vi "TURN_V2.vi"(0 "datain":string[](array[string])=["备注", "负载通道", "负载地址", "延时时间", "output max", "output min", "量测类型", "待测物板号"], 5 "HW CH Number":i32=4, 7 "Setup":string) -> (4 "REPORT INDECATE":string[][](array[string])=[["微安测试", "", "", "", ""], ["微安量测", "4", "0.000", "0.1", "NG"], ["微安量测", "4", "0.000", "0.1", "NG"], ["微安量测", "4", "0.000", "0.1", "NG"], ["微安量测", "4", "0.000", "0.1", "NG"]], 6 "ROW HEAD":string[](array[string]), 8 "PF":string[](array[string]), 10 "testData":string[](array[string]), 14 "数组":bool[](array[boolean]), 15 "Array":string[](array[string]))   [LabVIEW 2018]
uses:
  Subvi/Global.vi
panel:
  out "测试板数":i32=4
  # "[VoltageTest]\nExt.Name =2222222222;\nAddress =1;\nDelay Time =1;\nMAX.Spec =*;\nMin.Spec =2;\nTest Type =;\nRelayH_8Bit =0,0,0,0;\nRelayL_8Bit =0,0,0,0;\nStart board number =1;#"
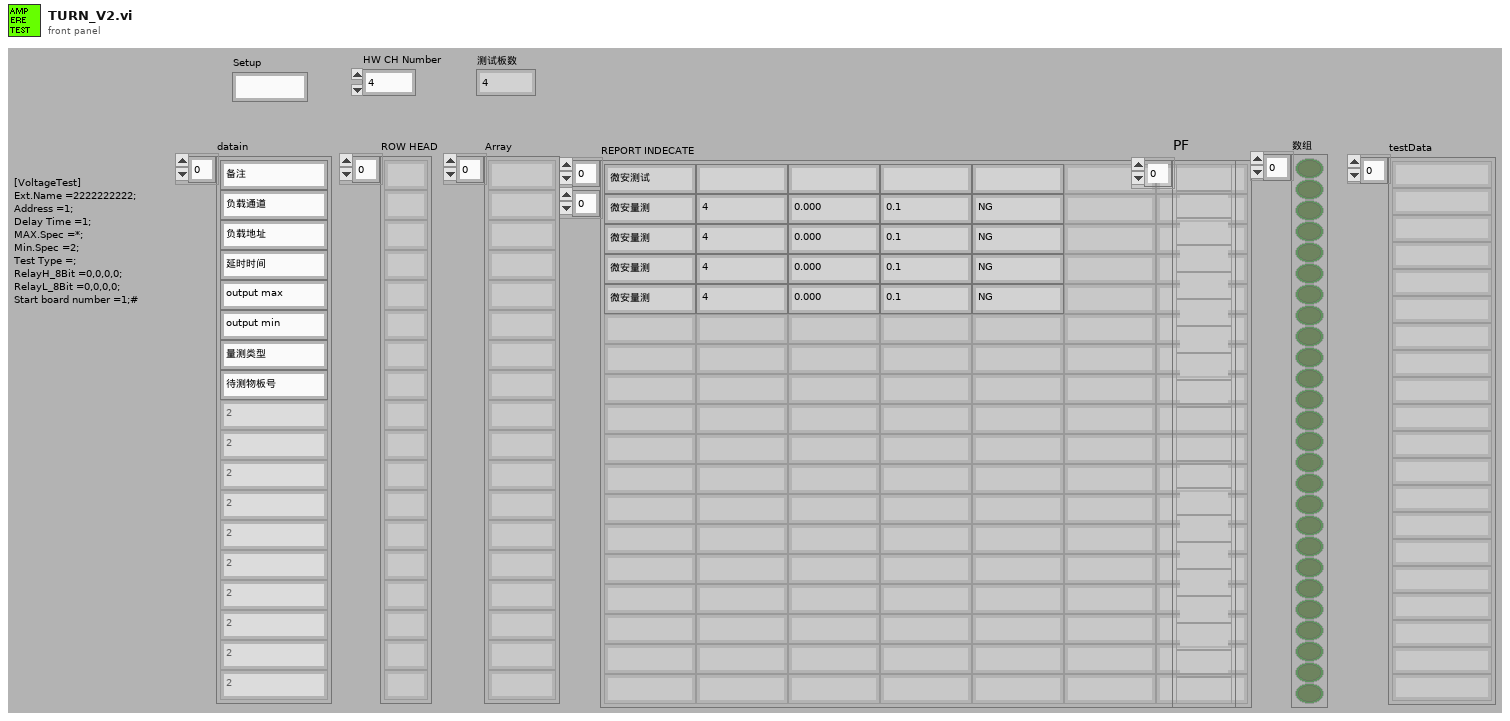
[diagram p1: front panel]
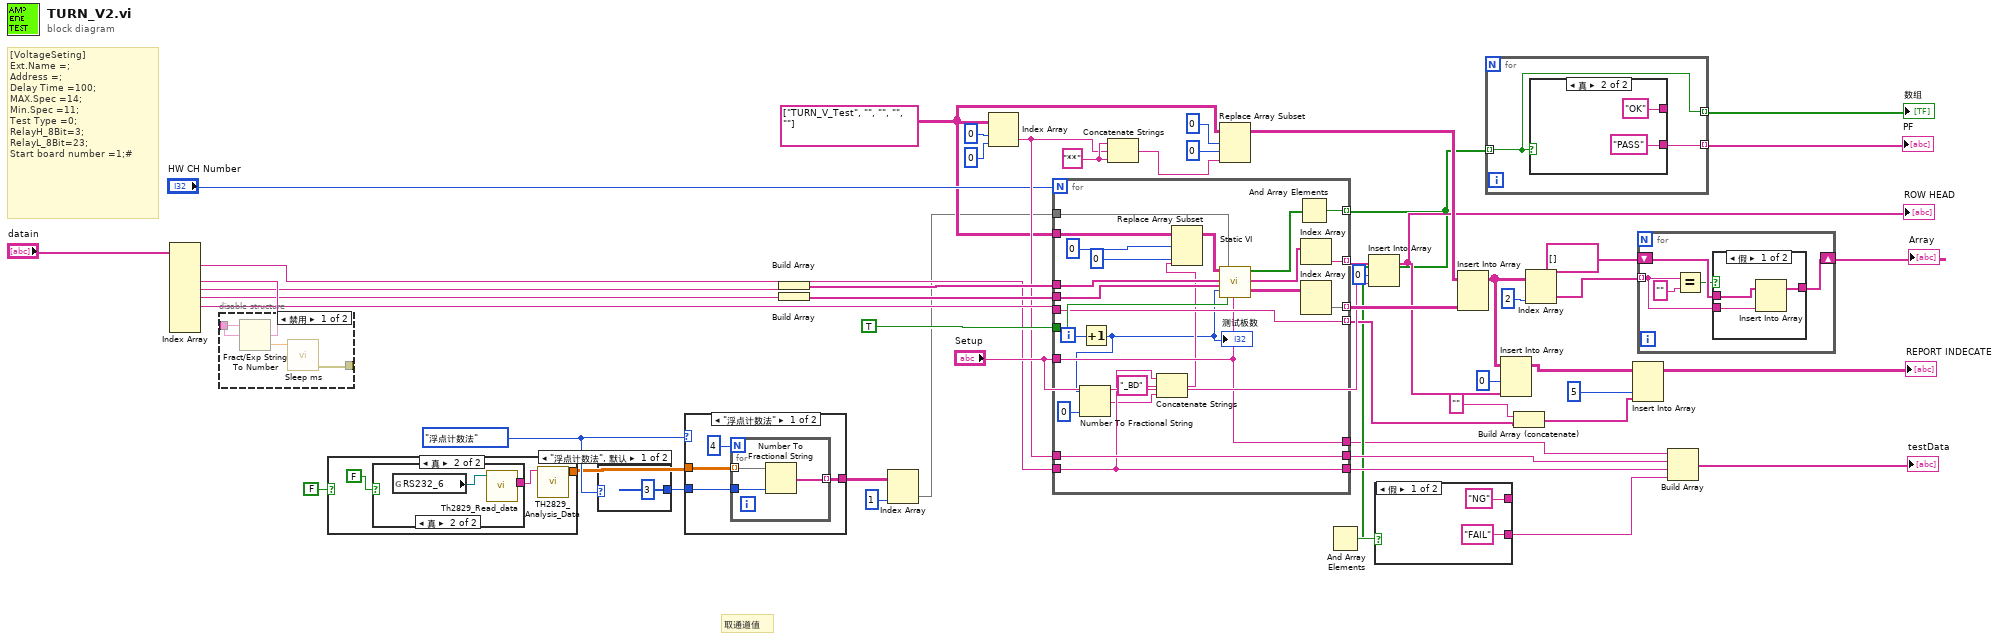
[diagram p0: block diagram]
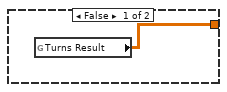
[diagram p2: hidden frame]
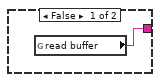
[diagram p3: hidden frame]
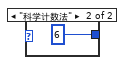
[diagram p4: hidden frame]
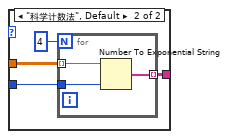
[diagram p5: hidden frame]
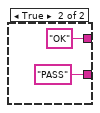
[diagram p7: hidden frame]
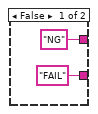
[diagram p8: hidden frame]
diagram:
  w6 = enum16{"浮点计数法", "科学计数法"}."浮点计数法" ("显示格式")
  w8 = string[][] [["TURN_V_Test", "", "", "", ""]]
  w43 = "**" ("字符串")
  # "取通道值"
  # "[VoltageSeting]\nExt.Name =;\nAddress =;\nDelay Time =100;\nMAX.Spec =14;\nMin.Spec =11;\nTest Type =0;\nRelayH_8Bit=3;\nRelayL_8Bit=23;\nStart board number =1;#"
  n1 = Index Array(array="datain") -> (element #1=w9:string, element #3=w46:string, element #4=w39:string, element #5=w38:string, element #6=w26:string)  [unwired: 9 in, 4 out]
  n2 = disable-structure shown="禁用" {
    disable-tunnel: w46 -> [w55 _]
    disable-tunnel: [w54 _] -> _
    frame Disabled {
      n3 = Fract/Exp String To Number(string=w55) -> (number=w53:dbl)  [unwired: 3 in, 1 out]
      n4 = call "Sleep ms.vi"("等待时间（毫秒）"=w53) -> ("error out"=w54:errorcluster)  [unwired: 10 in]
    }
    frame Enabled {
    }
  }
  n5 = case shown="真" FALSE {
    tunnel: [w56 w57] -> w5
    frame False {
      n6 = global read "Global.vi" "Turns Result"() -> (w56:sgl[][])
    }
    frame True {
      n7 = case shown="真" FALSE {
        tunnel: [w60 w62] -> w59
        frame False {
          n8 = global read "Global.vi" "read buffer"() -> (w60:string)
        }
        frame True {
          n9 = global read "Global.vi" "RS232_6"() -> (w61:refnum<visa-resource-name>)
          n10 = call "Th2829_Read_data.vi"("VISA资源名称"=w61) -> ("读取缓冲区"=w62:string)  [unwired: 9 in, 1 out]
        }
      }
      n11 = call "TH2829_Analysis_Data.vi"("字符串"=w59) -> ("Turns Result"=w57:sgl[][])  [unwired: 15 in, 3 out]
    }
  }
  n12 = case shown="\"浮点计数法\", 默认" w6 {
    tunnel: [i16 3 ("精度(6)") i16 6 ("精度(6)")] -> w7
    frame "浮点计数法", Default {
    }
    frame "科学计数法" {
    }
  }
  n13 = case shown="\"浮点计数法\"" w6 {
    tunnel: w5 -> [w67 w74]
    tunnel: [w66 w73] -> w4
    tunnel: w7 -> [w65 w72]
    frame "浮点计数法" {
      n14 = for {
        N: 4 -> [_]
        tunnel: w67 -> [w71] mode=indexing
        tunnel: [w70] -> w66 mode=indexing
        tunnel: w65 -> [w69]
        n15 = Number To Fractional String(number=w71, precision (6)=w69) -> (F-format string=w70:string[])  [unwired: 2 in]
      }
    }
    frame "科学计数法", Default {
      n16 = for {
        N: 4 -> [_]
        tunnel: w74 -> [w78] mode=indexing
        tunnel: [w77] -> w73 mode=indexing
        tunnel: w72 -> [w76]
        n17 = Number To Exponential String(number=w78, precision (6)=w76) -> (E-format string=w77:string[])  [unwired: 2 in]
      }
    }
  }
  n18 = Build Array(w39) -> (w37:string[])
  n19 = Build Array(w38) -> (w36:string[])
  n20 = Index Array(array=w4, index (col)=1 ("禁用的索引 (列)")) -> (element=w2:string[])  [unwired: 1 in]
  n21 = Index Array(array=w8, index (row)=0 ("索引 (行)"), index (col)=0 ("禁用的索引 (列)")) -> (element=w19:string)
  n22 = for {
    N: "HW CH Number" -> [_]
    tunnel: w2 -> [w102]
    tunnel: w37 -> [w101]
    tunnel: w36 -> [w100]
    tunnel: "Setup" -> [w90]
    tunnel: TRUE -> [w98]
    tunnel: [w97] -> w15 mode=indexing
    tunnel: [w95] -> w32 mode=indexing
    tunnel: [w93] -> w33 mode=indexing
    tunnel: w26 -> [w92]
    tunnel: [w92] -> w22 mode=indexing
    tunnel: w19 -> [w91]
    tunnel: [w91] -> w18
    tunnel: w9 -> [w82]
    tunnel: [w82] -> w17
    tunnel: [w90] -> w12
    tunnel: w8 -> [w88]
    i -> [w85]
    n23 = Increment(x=w85) -> (x+1=w79:i32)
    "测试板数" <- w79
    n24 = Number To Fractional String(number=w79, precision (6)=i16 0 ("精度(6)")) -> (F-format string=w81:string)  [unwired: 2 in]
    n25 = Concatenate Strings(w82, "_BD" ("字符串"), w81) -> (w80:string)
    n26 = Replace Array Subset(array=w88, new element=w80, index (row)=0 ("索引 (行)"), index (col)=0 ("禁用的索引 (列)")) -> (w87:string[][])
    n27 = call "Static VI.vi"("添加的数组"=w87, "Max"=w101, "Min"=w100, "板数"=w79, "INPUTSTRING"=w102, "是否为字符串对比"=w98, "SQ"=w90) -> ("P/F"=w99:bool[], "SQ out"=w96:string[], "arrauy out"=w94:string[][])  [unwired: 9 in, 1 out]
    n28 = And Array Elements(Boolean array=w99) -> (logical AND=w97:bool)
    n29 = Index Array(array=w96) -> (element=w95:string)  [unwired: 1 in]
    n30 = Index Array(array=w94) -> (element=w93:string[])  [unwired: 2 in]
  }
  n31 = Concatenate Strings(w43, w19, w43) -> (w40:string)
  n32 = Replace Array Subset(array=w8, new element=w40, index (row)=0 ("索引 (行)"), index (col)=0 ("禁用的索引 (列)")) -> (w34:string[][])
  n33 = And Array Elements(Boolean array=w15) -> (logical AND=w16:bool)
  n34 = Insert Into Array(array=w32, index=0 ("索引"), new element="Setup") -> (w28:string[])
  "ROW HEAD" <- w28
  n35 = case shown="假" w16 {
    tunnel: ["NG" "OK"] -> _
    tunnel: ["FAIL" "PASS"] -> w14
    frame False {
    }
    frame True {
    }
  }
  n36 = Insert Into Array ("数组插入")(array=w34, new element=w33) -> (w29:string[][])  [unwired: 2 in]
  n37 = for {
    tunnel: w15 -> [w107] mode=indexing
    tunnel: [w108] -> w48 mode=indexing
    tunnel: [w107] -> w11 mode=indexing
    n38 = case shown="真" w107 {
      tunnel: ["NG" "OK"] -> _
      tunnel: ["FAIL" "PASS"] -> w108
      frame False {
      }
      frame True {
      }
    }
  }
  "PF" <- w48
  "数组" <- w11
  n39 = Insert Into Array(array=w29, index (col)=0 ("禁用的索引 (列)"), new element=w28) -> (w24:string[][])  [unwired: 1 in]
  n40 = Build Array (concatenate)("" ("字符串"), w22) -> (w20:string[])
  n41 = Index Array(array=w29, index (col)=2 ("禁用的索引 (列)")) -> (element=w50:string[])  [unwired: 1 in]
  n42 = Insert Into Array(array=w24, index (col)=5 ("禁用的索引 (列)"), new element=w20) -> (→"REPORT INDECATE":string[][])  [unwired: 1 in]
  n43 = for {
    tunnel: w50 -> [w113] mode=indexing
    shift-right: [w114] -> w49
    shift-left: string[] [] ("Array") -> [w117]
    n44 = Equal?(x=w113, y="") -> (x = y?=w115:bool)
    n45 = case shown="假" w115 {
      tunnel: w117 -> [w120 w121]
      tunnel: [w119 w121] -> w114
      tunnel: w113 -> [w118 _]
      frame False {
        n46 = Insert Into Array(array=w120, new element=w118) -> (w119:string[])  [unwired: 1 in]
      }
      frame True {
      }
    }
  }
  "Array" <- w49
  n47 = Build Array(w12, w18, w17, w14) -> (→"testData":string[])
